vi "set_item_by_name.vi"(6 "close_item? (true)":bool=TRUE, 8 "error in":errorcluster, 9 "Item":refnum<class "Item.lvclass">, 10 "key_name":string, 11 "Table in":refnum<class "InlineTable.lvclass">) -> (0 "error out":errorcluster, 3 "Table out":refnum<class "InlineTable.lvclass">)   [LabVIEW 2020, in "toml_edit.lvlib" / "InlineTable.lvclass"]
uses:
  InlineTable.lvclass
  Item/Item.lvclass
  InlineTable.lvclass/InlineTable.ctl
  Item/Item.lvclass/Item.ctl
  dragon_toml_32.dll
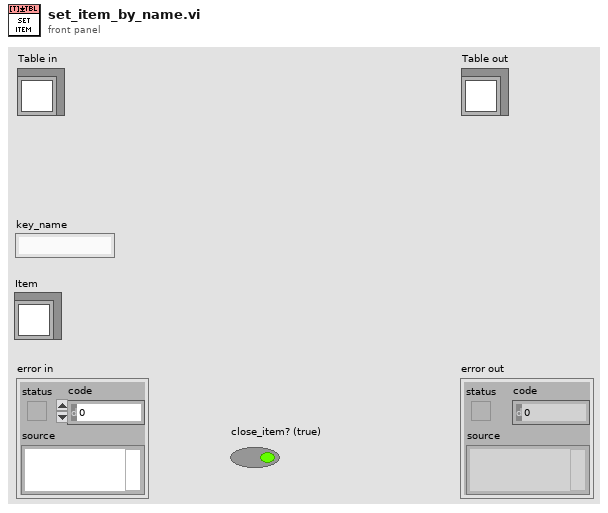
[diagram p1: front panel]
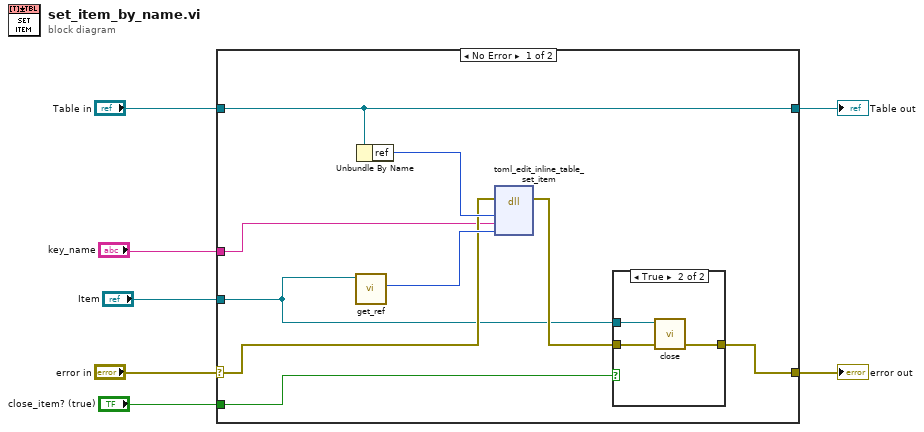
[diagram p0: block diagram]
diagram:
  n1 = case shown="No Error" "error in" {
    selector: "error in" -> [w13 w22]
    tunnel: [w11 w22] -> w6
    tunnel: [w10 w21] -> w4
    tunnel: "Table in" -> [w10 w21]
    tunnel: "key_name" -> [w9 _]
    tunnel: "Item" -> [w8 _]
    tunnel: "close_item? (true)" -> [w12 _]
    frame No Error {
      n2 = call "get_ref.vi"("Item in"=w8) -> ("ref"=w15:u64)  [unwired: 10 in]
      n3 = Unbundle By Name(w10) -> ("ref"=w14:u64)
      n4 = dll-call lib="C:/projects/dragon-desktop/source/submodules/toml-edit-labview/lv_src/dragon_toml_*.dll" fn="toml_edit_inline_table_set_item"(error in=w13, "table_ref"=w14, "item_name"=w9, "item_ref"=w15) -> (error out=w16:errorcluster)  [unwired: 6 in, 1 out]
      n5 = case shown="True" w12 {
        tunnel: w16 -> [w17 w20]
        tunnel: [w17 w19] -> w11
        tunnel: w8 -> [_ w18]
        frame False {
        }
        frame True {
          n6 = call "close.vi"("error in (no error)"=w20, "Item in"=w18) -> ("error out"=w19:errorcluster)  [unwired: 9 in]
        }
      }
    }
    frame Error {
    }
  }
  "error out" <- w6
  "Table out" <- w4
